vi "SveTDMS.vi"(5 "2D Array":dbl[][](array[numeric]), 6 "Serial Number":string="12358", 7 "Description":string="This is a TDMS file used in a LabVIEW Workshop", 8 "error in (no error)":errorcluster, 9 "Author":string="Calvek", 10 "Title":string="TorqueData", 11 "Path Control":path=path "C:/Users/Diego TURRUBIARTES/Desktop/prueba 719") -> (0 "error out":errorcluster)   [LabVIEW 2020]
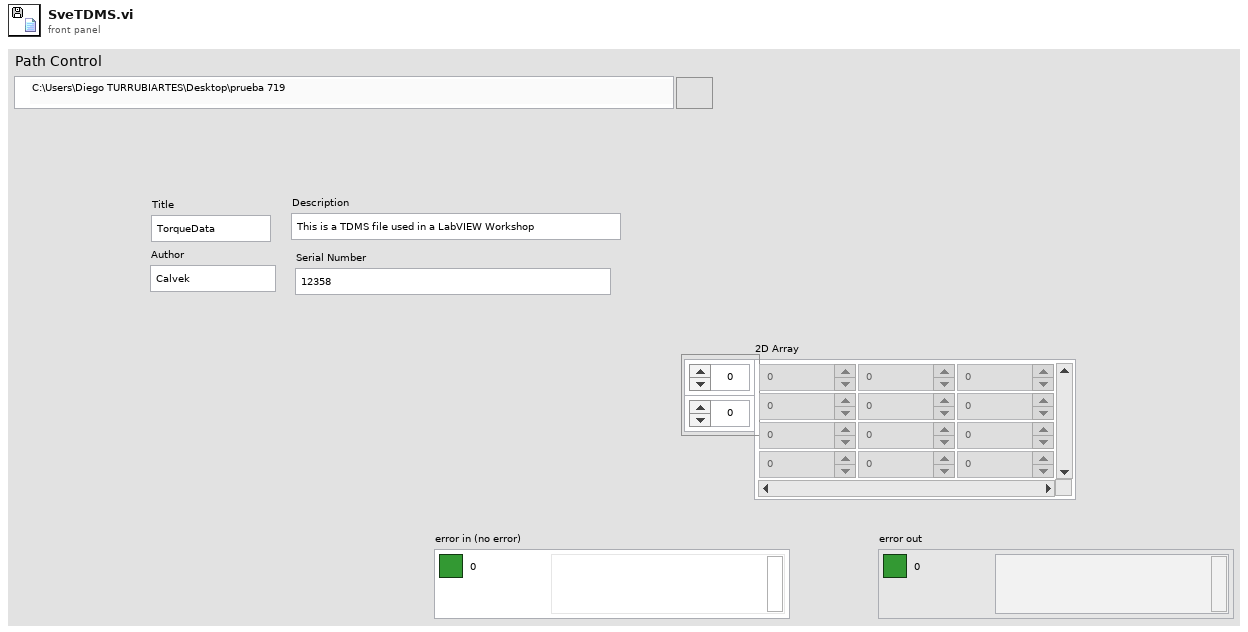
[diagram p1: front panel]
types:
  T1 = enum16{"open", "open or create", "create or replace", "create", "open (read-only)"}
  T2 = cluster{"Start Measure":bool, "Serial Number":string, "Delete Data":bool}
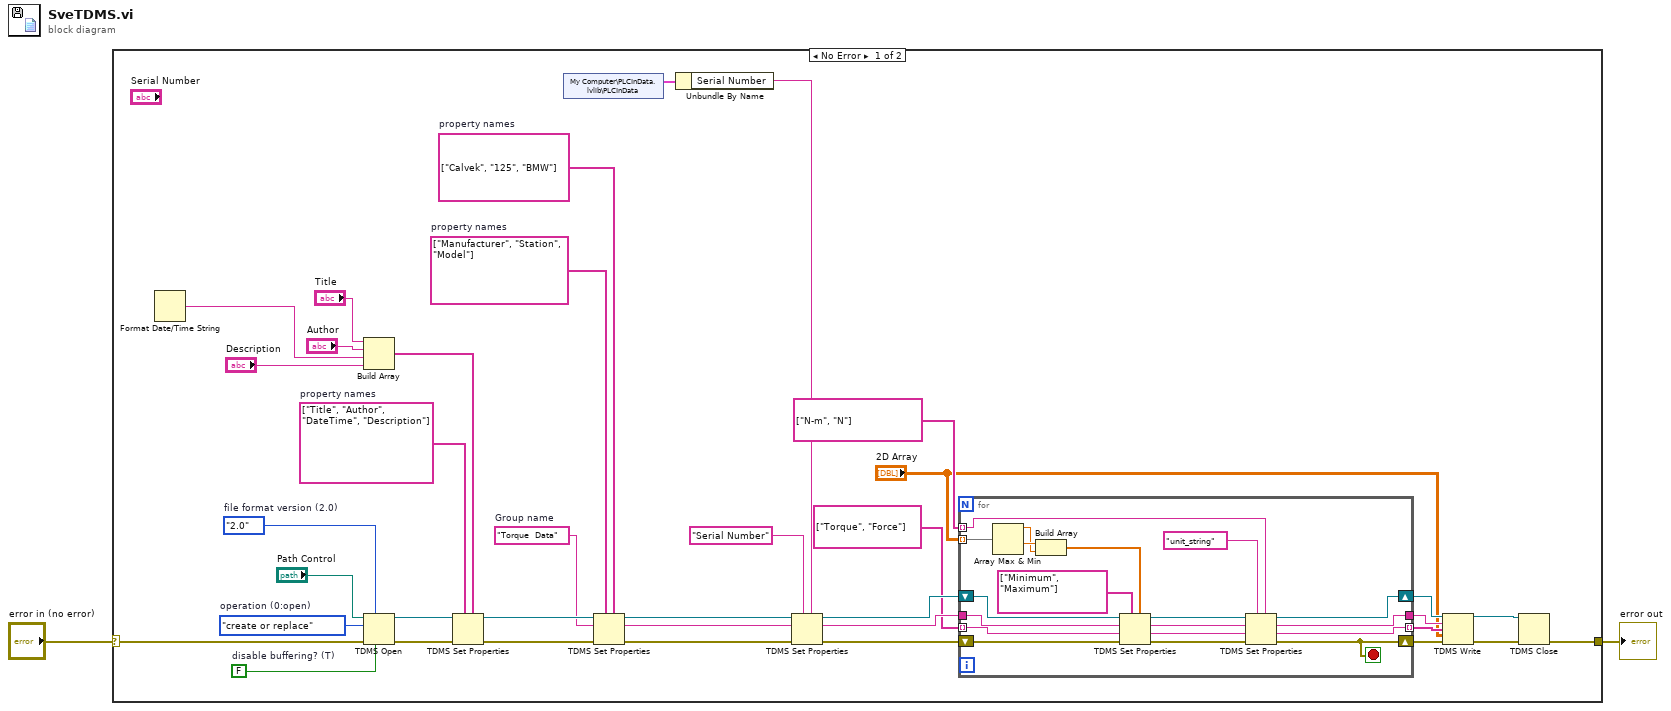
[diagram p0: block diagram]
diagram:
  n1 = case shown="No Error" "error in (no error)" {
    selector: "error in (no error)" -> [w19 w59]
    tunnel: [w27 w59] -> w1
    frame No Error {
      w34 = FALSE  # disable buffering? (T)
      w33 = enum16{"1.0", "2.0"}."2.0"  # file format version (2.0)
      w35 = T1."create or replace"  # operation (0:open)
      w37 = string[] ["Calvek", "125", "BMW"]  # property names
      w36 = string[] ["Manufacturer", "Station", "Model"]  # property names
      w29 = "Torque  Data"  # Group name
      w38 = string[] ["Title", "Author", "DateTime", "Description"]  # property names
      n2 = Format Date/Time String() -> (date/time string=w9:string)  [unwired: 3 in]
      n3 = Build Array "Build Array"("Title", "Author", w9, "Description") -> (w7:string[])
      n4 = TDMS Open(6:w34, 7:w33, 8:w19, 10:w35, 11:"Path Control") -> (0:w39:errorcluster, 3:w30:refnum<k34>)  [unwired: 2 in]
      n5 = TDMS Set Properties(5:w7, 7:w38, 8:w39, 11:w30) -> (0:w31:errorcluster, 3:w32:refnum<k34>)  [unwired: 2 in, 2 out]
      n6 = shared-variable "My Computer\\PLCInData.lvlib\\PLCInData"() -> (w4:T2)  [unwired: 1 in, 1 out]
      n7 = TDMS Set Properties(5:w37, 7:w36, 8:w31, 10:w29, 11:w32) -> (0:w26:errorcluster, 2:w24:string, 3:w25:refnum<k34>)  [unwired: 1 in, 1 out]
      n8 = Unbundle By Name "Unbundle By Name"(w4) -> ("Serial Number"=w3:string)
      n9 = TDMS Set Properties(5:w3, 7:"Serial Number", 8:w26, 10:w24, 11:w25) -> (0:w20:errorcluster, 2:w21:string, 3:w22:refnum<k34>)  [unwired: 1 in, 1 out]
      n10 = for {
        tunnel: string[] ["Torque", "Force"] -> [w54] mode=indexing
        tunnel: string[] ["N-m", "N"] -> [w53] mode=indexing
        tunnel: w21 -> [w50]
        shift-right: [w44] -> w17
        shift-left: w20 -> [w47]
        shift-right: [w48] -> w18
        shift-left: w22 -> [w49]
        tunnel: [w46] -> w16
        tunnel: [w45] -> w12 mode=indexing
        tunnel: "2D Array" -> [w43] mode=indexing
        stop <- w44 stop-if-true
        n11 = Array Max & Min(array=w43) -> (max value=w41:dbl, min value=w42:dbl)  [unwired: 2 out]
        n12 = Build Array(w42, w41) -> (w40:dbl[])
        n13 = TDMS Set Properties(5:w40, 7:string[] ["Minimum", "Maximum"] ("property names"), 8:w47, 9:w54, 10:w50, 11:w49) -> (0:w57:errorcluster, 1:w55:string, 2:w56:string, 3:w58:refnum<k34>)
        n14 = TDMS Set Properties(5:w53, 7:"unit_string", 8:w57, 9:w55, 10:w56, 11:w58) -> (0:w44:errorcluster, 1:w45:string, 2:w46:string, 3:w48:refnum<k34>)
      }
      n15 = TDMS Write(0:w18, 5:w16, 7:w12, 9:"2D Array", 11:w17) -> (4:w15:refnum<k34>, 15:w14:errorcluster)  [unwired: 1 in, 2 out]
      n16 = TDMS Close(8:w14, 11:w15) -> (0:w27:errorcluster)  [unwired: 1 out]
    }
    frame Error {
    }
  }
  "error out" <- w1
